vi "Write CurrName.vi"(8 "error in (no error)":errorcluster, 10 "CurrName":u8[](array[numeric]), 11 "HighscoreDialog in":refnum<class "HighscoreDialog.lvclass">) -> (0 "error out":errorcluster, 3 "HighscoreDialog out":refnum<class "HighscoreDialog.lvclass">)   [LabVIEW 2019, in "RT_Game.lvlib" / "HighscoreDialog.lvclass"]
uses:
  HighscoreDialog.lvclass
  HighscoreDialog.lvclass/HighscoreDialog.ctl
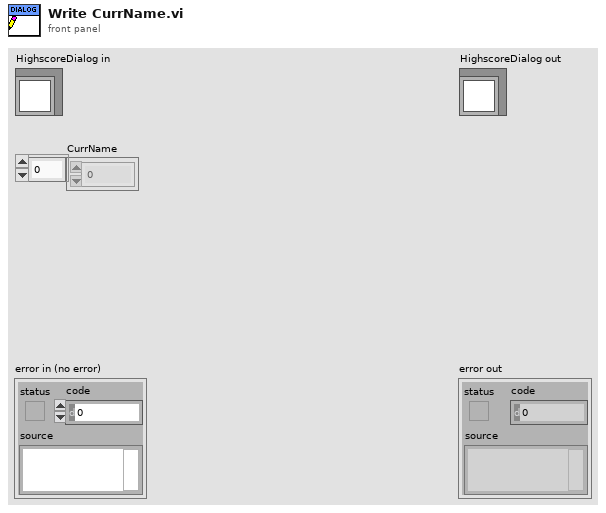
[diagram p1: front panel]
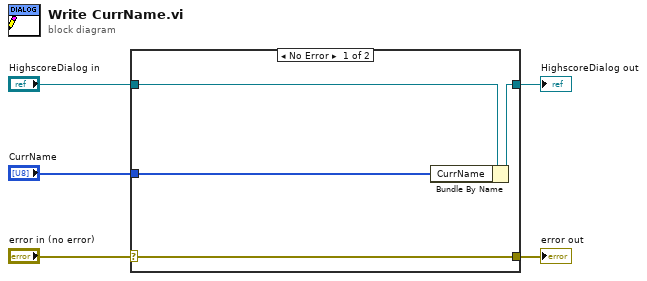
[diagram p0: block diagram]
diagram:
  n1 = case shown="No Error" "error in (no error)" {
    selector: "error in (no error)" -> [w9 w10]
    tunnel: [w9 w10] -> w4
    tunnel: [w7 w11] -> w2
    tunnel: "HighscoreDialog in" -> [w8 w11]
    tunnel: "CurrName" -> [w6 _]
    frame No Error {
      n2 = Bundle By Name(cluster=w8, "CurrName"=w6) -> (w7:refnum<class "HighscoreDialog.lvclass">)
    }
    frame Error {
    }
  }
  "error out" <- w4
  "HighscoreDialog out" <- w2
